vi "solar_type Variant to Arguments.vi"(2 "Variant":variant) -> (7 "Value1, Value2...":string)   [LabVIEW 2018]
doc: "This unpacks the variant into comma delimited ASCII values. This is used to record the SOLAR log data in human readable values."
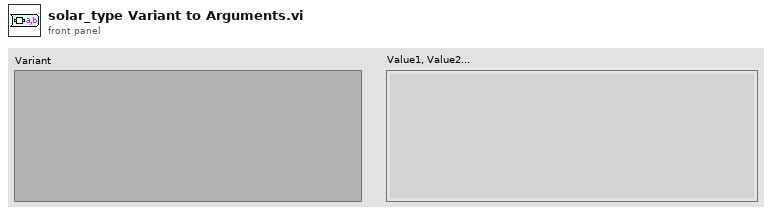
[diagram p1: front panel]
types:
  T1 = typedef "solar_type Item.ctl" = cluster{"Item":string, "Type":T2, "Value":variant, "States":string[]}
  T2 = typedef "solar_type Item Type.ctl" = enum16{"NULL", "UNKNOWN", "CLUSTER", "I8", "I16", "I32", "I64", "U8", "U16", "U32", "U64", "U8_ENUM", "U16_ENUM", "U32_ENUM", "SGL", "DBL", "BOOLEAN", "STRING", "PATH", "VISA", "TAG", "TIME", "I8_1D", "I16_1D", "I32_1D", "I64_1D", "U8_1D", "U16_1D", "U32_1D", "U64_1D", "U8_ENUM_1D", "U16_ENUM_1D", "U32_ENUM_1D", "SGL_1D", "DBL_1D", "BOOLEAN_1D", "STRING_1D", "PATH_1D", "VISA_1D", "TAG_1D", "TIME_1D", "I8_2D", "I16_2D", "I32_2D", "I64_2D", "U8_2D", "U16_2D", "U32_2D", "U64_2D", "U8_ENUM_2D", "U16_ENUM_2D", "U32_ENUM_2D", "SGL_2D", "DBL_2D", "BOOLEAN_2D", "STRING_2D", "PATH_2D", "VISA_2D", "TAG_2D", "TIME_2D"}
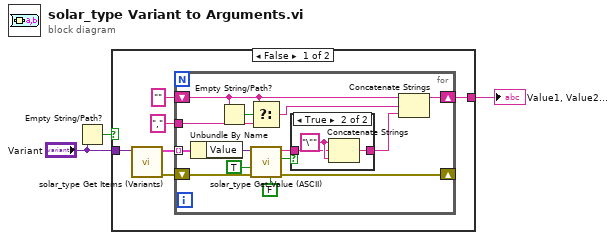
[diagram p0: block diagram]
diagram:
  n1 = Empty String/Path?(string/path="Variant") -> (empty?=w1:bool)
  n2 = case shown="False" w1 {
    tunnel: "Variant" -> [w6 _]
    tunnel: [w7 _] -> w3
    frame False {
      n3 = call "solar_type Get Items (Variants).vi"("Variant"=w6) -> ("error out"=w4:errorcluster, "Items"=w5:T1[])  [unwired: 7 in, 2 out]
      n4 = for {
        shift-right: [w23] -> w7
        shift-left: "" -> [w21]
        tunnel: "," -> [w20]
        shift-right: [w14] -> _
        shift-left: w4 -> [w18]
        tunnel: w5 -> [w17] mode=indexing
        n5 = Unbundle By Name(w17) -> ("Value"=w16:variant)
        n6 = Empty String/Path?(string/path=w21) -> (empty?=w22:bool)
        n7 = Select(t=w21, s=w22, f=w20) -> (s? t:f=w19:string)
        n8 = call "solar_type Get Value (ASCII).vi"("Boolean as 0,1? (F)"=FALSE, "error in (no error)"=w18, "Use Enum Names? (F)"=TRUE, "Variant"=w16) -> ("error out"=w14:errorcluster, "Quotes Recommended?"=w10:bool, "Value (ASCII)"=w12:string)  [unwired: 5 in]
        n9 = case shown="True" w10 {
          tunnel: w12 -> [w24 w26]
          tunnel: [w24 w25] -> w11
          frame False {
          }
          frame True {
            w27 = "\"" ("string")
            n10 = Concatenate Strings(w27, w26, w27) -> (w25:string)
          }
        }
        n11 = Concatenate Strings(w21, w19, w11) -> (w23:string)
      }
    }
    frame True {
    }
  }
  "Value1, Value2..." <- w3
